vi "Render.vi"(11 "Game Board in":refnum<class "Game Board.lvclass">) -> (2 "game Board":u32[][](array[colorbox]), 3 "Game Board out":refnum<class "Game Board.lvclass">)   [LabVIEW 2020, in "Game Board.lvclass"]
uses:
  Game Board.lvclass
  Game Board.lvclass/Game Board.ctl
  Drawable/Drawable.lvclass
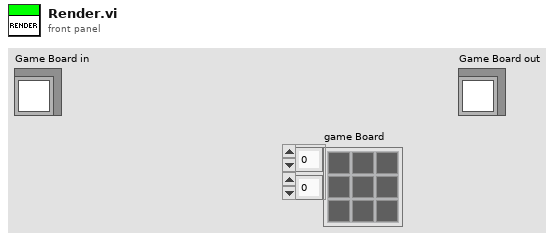
[diagram p1: front panel]
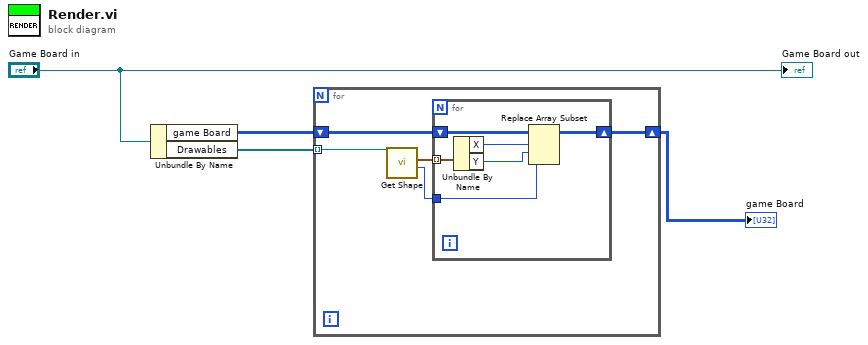
[diagram p0: block diagram]
diagram:
  n1 = Unbundle By Name("Game Board in") -> ("game Board"=w2:u32[][], "Drawables"=w3:refnum<class "Drawable.lvclass">[])
  n2 = for {
    tunnel: w3 -> [w9] mode=indexing
    shift-right: [w7] -> w1
    shift-left: w2 -> [w8]
    n3 = call-dynamic "Get Shape.vi"("Drawable in"=w9) -> ("Color"=w5:u32, "Coordinates"=w6:cluster{"X":i32, "Y":i32}[])  [unwired: 8 in, 1 out]
    n4 = for {
      tunnel: w6 -> [w13] mode=indexing
      shift-right: [w14] -> w7
      shift-left: w8 -> [w15]
      tunnel: w5 -> [w10]
      n5 = Unbundle By Name(w13) -> ("X"=w12:i32, "Y"=w11:i32)
      n6 = Replace Array Subset(array=w15, new element=w10, index (row)=w12, index (col)=w11) -> (w14:u32[][])
    }
  }
  "game Board" <- w1
  "Game Board out" <- "Game Board in"
